vi "Read Auto-open.vi"(8 "error in (no error)":errorcluster, 11 "Mag Lab Measure UI in":refnum<class "Mag Lab Measure UI.lvclass">) -> (0 "error out":errorcluster, 2 "Auto-open":bool, 3 "Mag Lab Measure UI out":refnum<class "Mag Lab Measure UI.lvclass">)   [LabVIEW 2015, in "Mag Lab Measure UI.lvclass"]
uses:
  Mag Lab Measure UI.lvclass
  Mag Lab Measure UI.lvclass/Mag Lab Measure UI.ctl
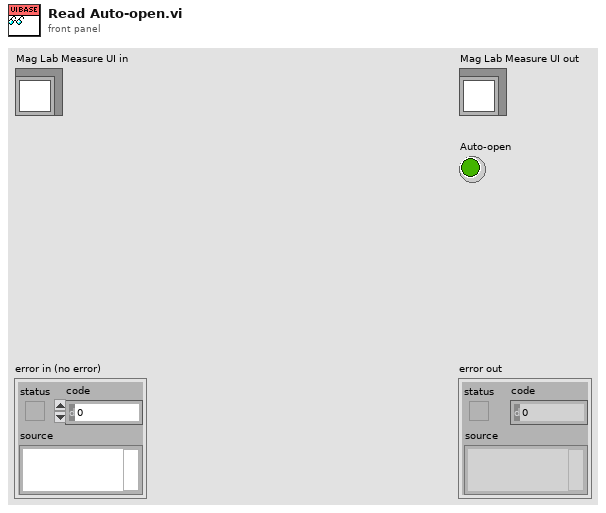
[diagram p1: front panel]
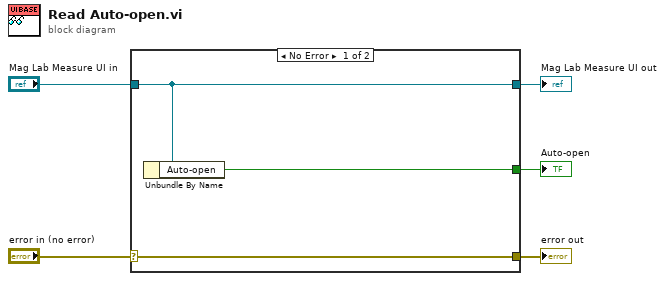
[diagram p0: block diagram]
diagram:
  n1 = case shown="No Error" "error in (no error)" {
    selector: "error in (no error)" -> [w8 w9]
    tunnel: [w8 w9] -> w4
    tunnel: [w7 w10] -> w2
    tunnel: "Mag Lab Measure UI in" -> [w7 w10]
    tunnel: [w6 _] -> w1
    frame No Error {
      n2 = Unbundle By Name(w7) -> ("Auto-open"=w6:bool)
    }
    frame Error {
    }
  }
  "error out" <- w4
  "Mag Lab Measure UI out" <- w2
  "Auto-open" <- w1
